vi "测试报告_1.vi"() -> ()   [LabVIEW 2010]
uses:
  <vilib>/Utility/NIReport.llb/NI_report.lvclass
  全局量/自动测试结果.vi
  全局量/试验配置信息.vi
  <vilib>/addons/_office/word.llb/Word Easy Table (str).vi
  <vilib>/addons/_office/NI_ReportGenerationToolkit.lvlib
panel:
  out "XY图":cluster{"Y":dbl[], "Y":dbl[]}[](graph)
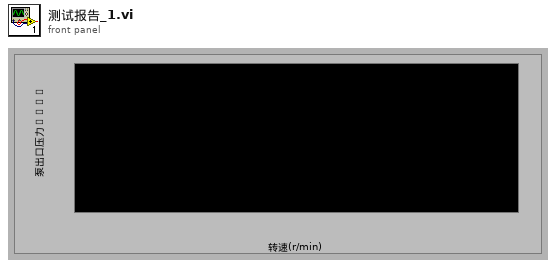
[diagram p1: front panel]
types:
  T1 = enum16{"maximized", "minimized", "normal", "no change"}
  T2 = enum16{"Standard Report", "HTML", "Word", "Excel"}
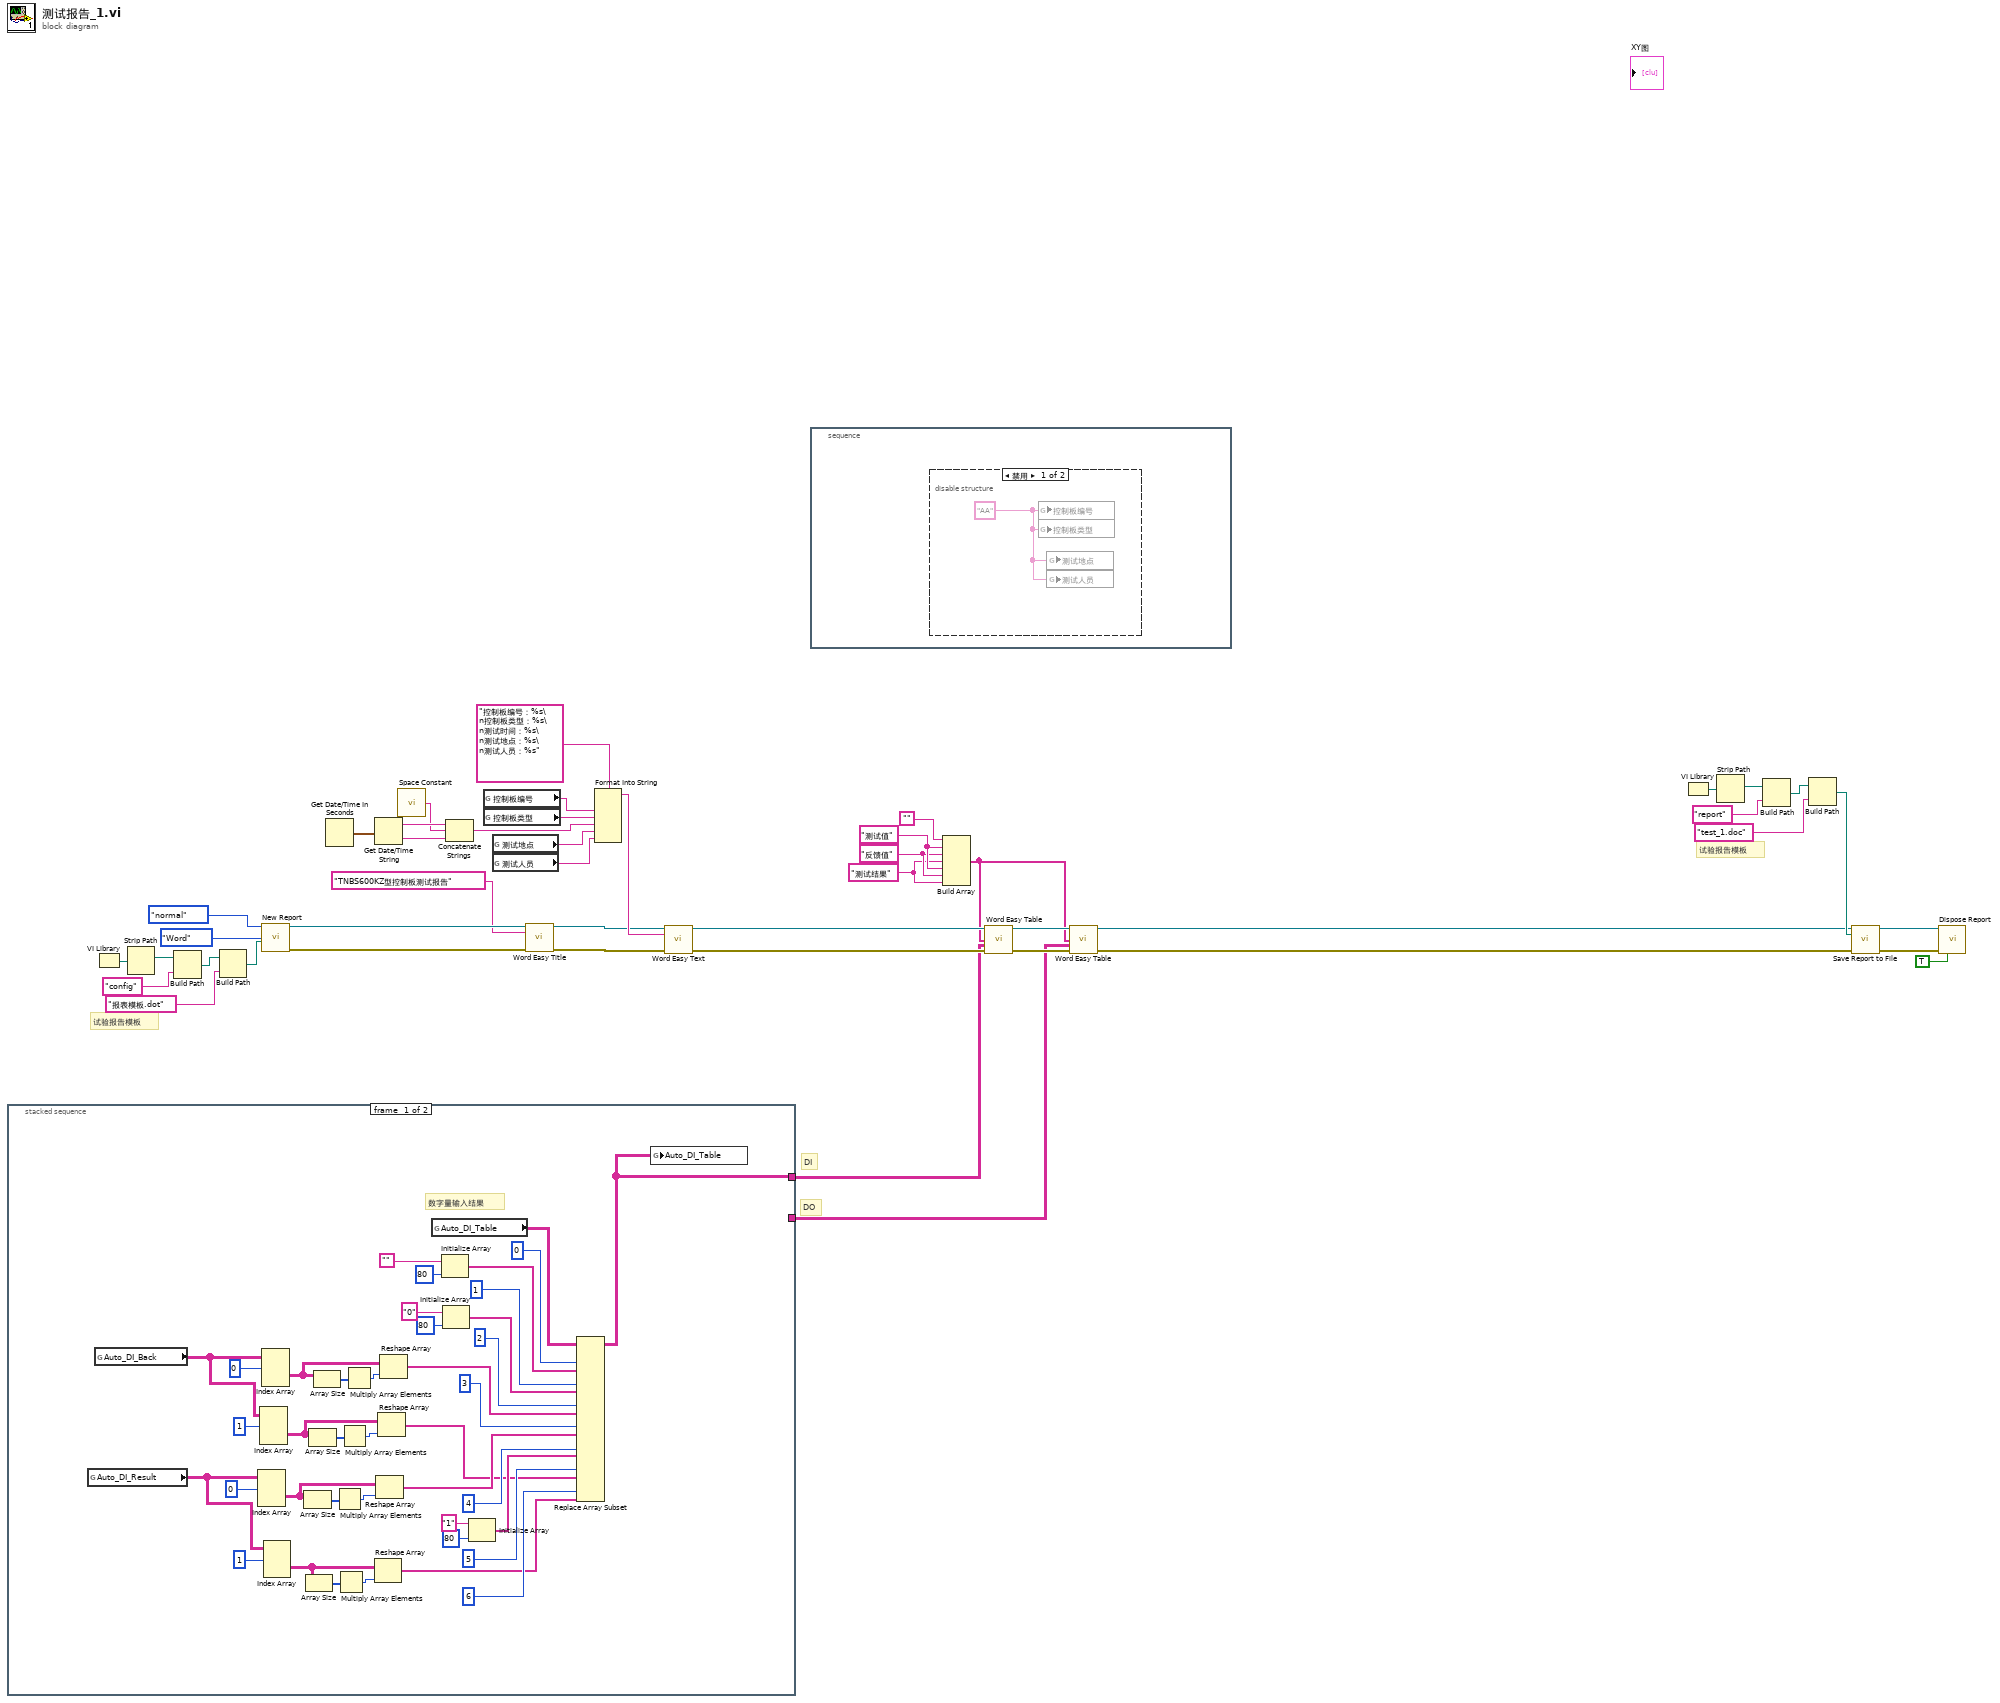
[diagram p0: block diagram]
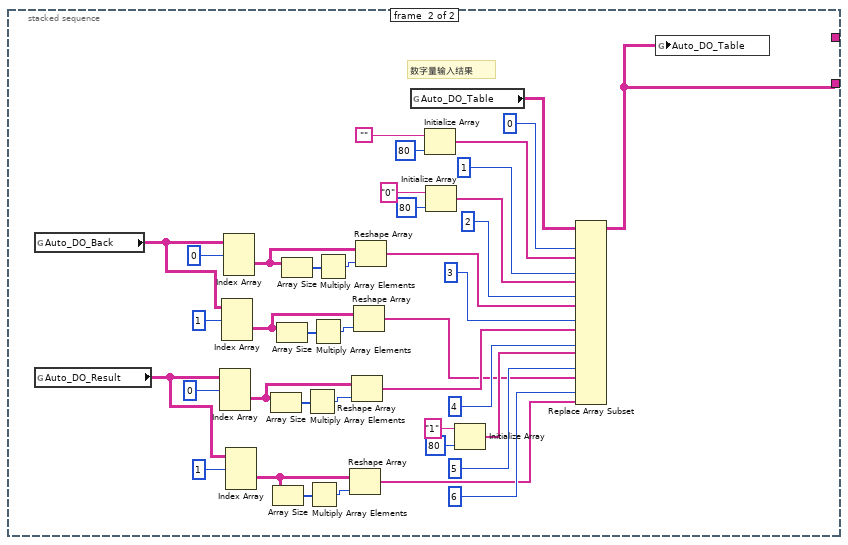
[diagram p3: hidden frame]
diagram:
  w15 = "测试结果"
  w16 = "反馈值"
  w17 = "测试值"
  # "DO"
  # "DI"
  # "试验报告模板"
  # "试验报告模板"
  n1 = stacked-sequence {
    tunnel: [w47 _] -> w7
    tunnel: [_ w87] -> w6
    frame #0 {
      # "数字量输入结果"
      n2 = global read "自动测试结果.vi" "Auto_DI_Result"() -> (w77:string[][][])
      n3 = global read "自动测试结果.vi" "Auto_DI_Back"() -> (w69:string[][][])
      n4 = Index Array(array=w77, index (dim 0)=0 ("索引 (页)")) -> (element=w82:string[][])  [unwired: 2 in]
      n5 = Index Array(array=w69, index (dim 0)=1 ("索引 (页)")) -> (element=w65:string[][])  [unwired: 2 in]
      n6 = Index Array(array=w69, index (dim 0)=0 ("索引 (页)")) -> (element=w64:string[][])  [unwired: 2 in]
      n7 = Index Array(array=w77, index (dim 0)=1 ("索引 (页)")) -> (element=w81:string[][])  [unwired: 2 in]
      n8 = Array Size(array=w82) -> (size(s)=w84:i32[])
      n9 = Array Size(array=w81) -> (size(s)=w79:i32[])
      n10 = Array Size(array=w65) -> (size(s)=w67:i32[])
      n11 = Array Size(array=w64) -> (size(s)=w62:i32[])
      n12 = Multiply Array Elements(1:w84) -> (0:w83:i32)
      n13 = Multiply Array Elements(1:w79) -> (0:w80:i32)
      n14 = Multiply Array Elements(1:w67) -> (0:w66:i32)
      n15 = Multiply Array Elements(1:w62) -> (0:w63:i32)
      n16 = Reshape Array(w81, w80) -> (w49:string[])
      n17 = Reshape Array(w82, w83) -> (w57:string[])
      n18 = Reshape Array(w65, w66) -> (w51:string[])
      n19 = Reshape Array(w64, w63) -> (w59:string[])
      n20 = global read "自动测试结果.vi" "Auto_DI_Table"() -> (w86:string[][])
      n21 = Initialize Array("", 80 ("维数大小")) -> (w70:string[])
      n22 = Initialize Array("0", 80 ("维数大小")) -> (w72:string[])
      n23 = Initialize Array("1", 80 ("维数大小")) -> (w53:string[])
      n24 = Replace Array Subset(array=w86, new element #1=w70, index (col) #1=0 ("禁用的索引 (列)"), new element #2=w72, index (col) #2=1 ("禁用的索引 (列)"), new element #3=w59, index (col) #3=2 ("禁用的索引 (列)"), new element #4=w57, index (col) #4=3 ("禁用的索引 (列)"), new element #5=w53, index (col) #5=4 ("禁用的索引 (列)"), new element #6=w51, index (col) #6=5 ("禁用的索引 (列)"), new element #7=w49, index (col) #7=6 ("禁用的索引 (列)")) -> (w47:string[][])  [unwired: 7 in]
      n25 = global write "自动测试结果.vi" "Auto_DI_Table"(w47) -> ()
    }
    frame #1 {
      # "数字量输入结果"
      n26 = global read "自动测试结果.vi" "Auto_DO_Back"() -> (w109:string[][][])
      n27 = global read "自动测试结果.vi" "Auto_DO_Result"() -> (w117:string[][][])
      n28 = Index Array(array=w117, index (dim 0)=0 ("索引 (页)")) -> (element=w122:string[][])  [unwired: 2 in]
      n29 = Index Array(array=w109, index (dim 0)=1 ("索引 (页)")) -> (element=w105:string[][])  [unwired: 2 in]
      n30 = Index Array(array=w109, index (dim 0)=0 ("索引 (页)")) -> (element=w104:string[][])  [unwired: 2 in]
      n31 = Index Array(array=w117, index (dim 0)=1 ("索引 (页)")) -> (element=w121:string[][])  [unwired: 2 in]
      n32 = Array Size(array=w122) -> (size(s)=w124:i32[])
      n33 = Array Size(array=w121) -> (size(s)=w119:i32[])
      n34 = Array Size(array=w105) -> (size(s)=w107:i32[])
      n35 = Array Size(array=w104) -> (size(s)=w102:i32[])
      n36 = Multiply Array Elements(1:w124) -> (0:w123:i32)
      n37 = Multiply Array Elements(1:w119) -> (0:w120:i32)
      n38 = Multiply Array Elements(1:w107) -> (0:w106:i32)
      n39 = Multiply Array Elements(1:w102) -> (0:w103:i32)
      n40 = Reshape Array(w121, w120) -> (w89:string[])
      n41 = Reshape Array(w122, w123) -> (w97:string[])
      n42 = Reshape Array(w105, w106) -> (w91:string[])
      n43 = Reshape Array(w104, w103) -> (w99:string[])
      n44 = global read "自动测试结果.vi" "Auto_DO_Table"() -> (w126:string[][])
      n45 = Initialize Array("", 80 ("维数大小")) -> (w110:string[])
      n46 = Initialize Array("0", 80 ("维数大小")) -> (w112:string[])
      n47 = Initialize Array("1", 80 ("维数大小")) -> (w93:string[])
      n48 = Replace Array Subset(array=w126, new element #1=w110, index (col) #1=0 ("禁用的索引 (列)"), new element #2=w112, index (col) #2=1 ("禁用的索引 (列)"), new element #3=w99, index (col) #3=2 ("禁用的索引 (列)"), new element #4=w97, index (col) #4=3 ("禁用的索引 (列)"), new element #5=w93, index (col) #5=4 ("禁用的索引 (列)"), new element #6=w91, index (col) #6=5 ("禁用的索引 (列)"), new element #7=w89, index (col) #7=6 ("禁用的索引 (列)")) -> (w87:string[][])  [unwired: 7 in]
      n49 = global write "自动测试结果.vi" "Auto_DO_Table"(w87) -> ()
    }
  }
  n50 = VI Library() -> (path=w42:path)
  n51 = Strip Path(path=w42) -> (stripped path=w45:path)  [unwired: 1 out]
  n52 = Build Path(base path=w45, name or relative path="config") -> (appended path=w43:path)
  n53 = Build Path(base path=w43, name or relative path="报表模板.dot") -> (appended path=w30:path)
  n54 = call <vilib>:"New Report.vi"("window state (normal)"=T1."normal", "report type"=T2."Word", "template (empty)"=w30) -> ("report out"=w5:refnum<class "NI_report.lvclass">, "error out"=w4:errorcluster)  [unwired: 11 in]
  n55 = Get Date/Time In Seconds() -> (seconds since 1Jan1904=w28:timestamp)
  n56 = Get Date/Time String(seconds (now)=w28) -> (date string=w27:string, time string=w26:string)  [unwired: 2 in]
  n57 = call <vilib>:"Space Constant.vi"() -> ("String"=w25:string)
  n58 = Concatenate Strings(w27, w25, w26) -> (w22:string)
  n59 = global read "试验配置信息.vi" "控制板编号"() -> (w24:string)
  n60 = global read "试验配置信息.vi" "控制板类型"() -> (w23:string)
  n61 = global read "试验配置信息.vi" "测试地点"() -> (w21:string)
  n62 = global read "试验配置信息.vi" "测试人员"() -> (w20:string)
  n63 = call <vilib>:"Word Easy Title.vi"("report in"=w5, "title"="TNBS600KZ型控制板测试报告", "error in (no error)"=w4) -> ("report out"=w2:refnum<class "NI_report.lvclass">, "error out"=w3:errorcluster)  [unwired: 10 in, 1 out]
  n64 = Format Into String(format string="控制板编号：%s\n控制板类型：%s\n测试时间：%s\n测试地点：%s\n测试人员：%s", w24, w23, w22, w21, w20) -> (resulting string=w19:string)  [unwired: 2 in, 1 out]
  n65 = call <vilib>:"Word Easy Text.vi"("report in"=w2, "text"=w19, "error in (no error)"=w3) -> ("report out"=w14:refnum<class "NI_report.lvclass">, "error out"=w13:errorcluster)  [unwired: 10 in, 1 out]
  n66 = stacked-sequence {
    frame #0 {
      n67 = disable-structure shown="禁用" {
        frame Disabled {
          w127 = "AA" ("控制板编号")
          n68 = global write "试验配置信息.vi" "控制板编号"(w127) -> ()
          n69 = global write "试验配置信息.vi" "控制板类型"(w127) -> ()
          n70 = global write "试验配置信息.vi" "测试地点"(w127) -> ()
          n71 = global write "试验配置信息.vi" "测试人员"(w127) -> ()
        }
        frame Enabled {
        }
      }
    }
  }
  n72 = Build Array("", w17, w16, w15, w17, w16, w15) -> (w8:string[])
  n73 = call-poly <vilib>:"Word Easy Table.vi"("report in"=w14, "column headers"=w8, "data"=w7, "error in (no error)"=w13) -> ("report out"=w12:refnum<class "NI_report.lvclass">, "error out"=w11:errorcluster)  [unwired: 9 in, 1 out]
  n74 = call-poly <vilib>:"Word Easy Table.vi"("report in"=w12, "column headers"=w8, "data"=w6, "error in (no error)"=w11) -> ("report out"=w10:refnum<class "NI_report.lvclass">, "error out"=w9:errorcluster)  [unwired: 9 in, 1 out]
  n75 = VI Library() -> (path=w32:path)
  n76 = Strip Path(path=w32) -> (stripped path=w35:path)  [unwired: 1 out]
  n77 = Build Path(base path=w35, name or relative path="report") -> (appended path=w33:path)
  n78 = Build Path(base path=w33, name or relative path="test_1.doc") -> (appended path=w37:path)
  n79 = call-dynamic "Save Report to File.vi"("report in"=w10, "report file path"=w37, "error in (no error)"=w9) -> ("report out"=w38:refnum<class "NI_report.lvclass">, "error out"=w39:errorcluster)  [unwired: 11 in]
  n80 = call-dynamic "Dispose Report.vi"("report in"=w38, "error in (no error)"=w39, "close report? (T)"=TRUE) -> ()  [unwired: 12 in, 1 out]
